vi "GetProcessInstanceRef.vi"(8 "error in (no error)":errorcluster, 10 "Process Name":string, 11 "JKI SMO in":refnum<class "JKI SMO.lvclass">) -> (0 "error out":errorcluster, 2 "Process VI Refnum":refnum<vi>, 3 "JKI SMO out":refnum<class "JKI SMO.lvclass">)   [LabVIEW 2013, in "JKI SMO.lvclass"]
doc: "This method will lookup (and return) the instance reference of <b>Process Name</b>.\n\n---------------------------------------------------------------\nJKI State Machine Objects™\nhttp://jki.net/state-machine-objects/\nCopyright (C) 2005-2015, JKI <info@jki.net>\nALL RIGHTS RESERVED"
uses:
  JKI SMO.lvclass
  JKI SMO.lvclass/JKI SMO.ctl
panel:
  # "For instructions on how to use the JKI State Machine Objects, examples and video tutorials, visit:\nhttp://jki.net/state-machine-objects/\n\nJKI State Machine Objects™\nhttp://jki.net/state-machine-objects/\nCopyright (C) 2005-2015, JKI <info@jki.net>\nALL RIGHTS RESERVED"
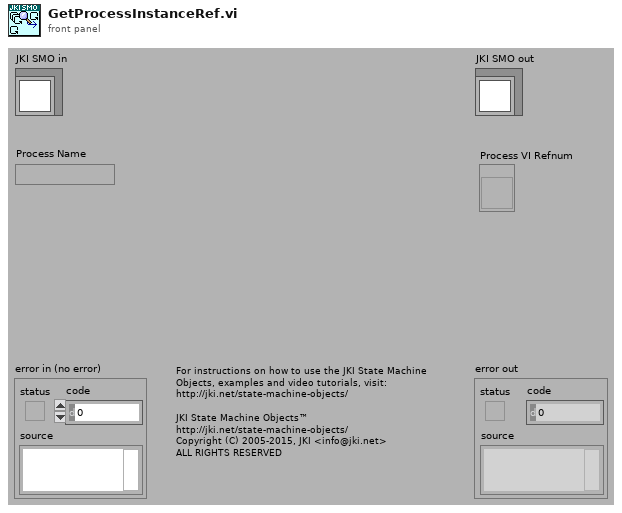
[diagram p1: front panel]
types:
  T1 = typedef "JKI SMO.lvclass/PrivateData--Cluster.ctl" = cluster{"Processes Clone VI Ref [ ]":refnum<vi>[], "Processes Clone Name [ ]":string[], "Process Sync RendezVous":T2, "Protected Events":T3, "Registered Process [ ]":T4[]}
  T2 = typedef "Rendezvous RefNum" = refnum<k1>
  T3 = typedef "JKI SMO.lvclass/ProtectedEvents--Cluster.ctl" = cluster{"StopProcesses":refnum<user-event>, "AbortProcesses":refnum<user-event>}
  T4 = typedef "JKI SMO.lvclass/RegisteredProcessData--Cluster.ctl" = cluster{"Name":string, "Static VI Ref":refnum<vi>}
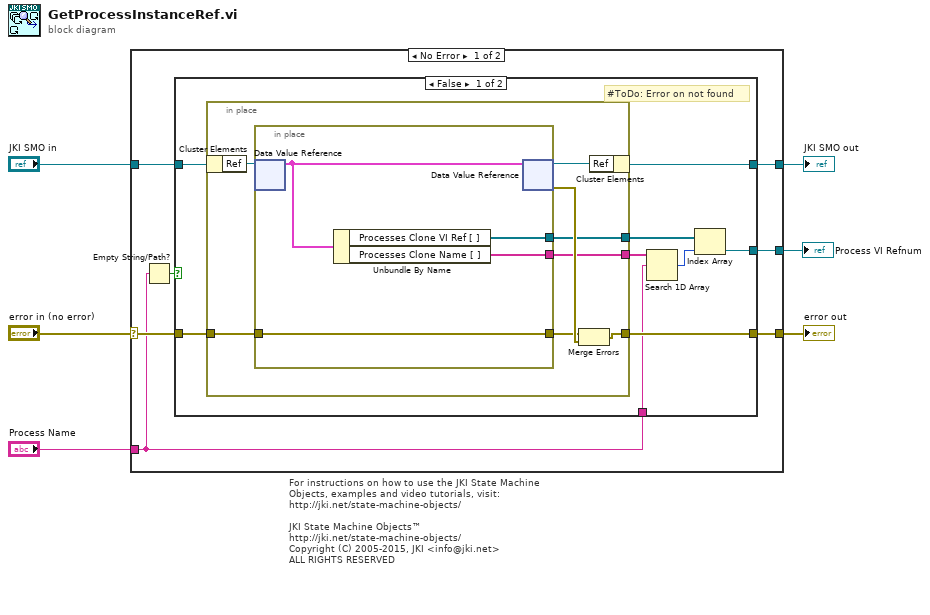
[diagram p0: block diagram]
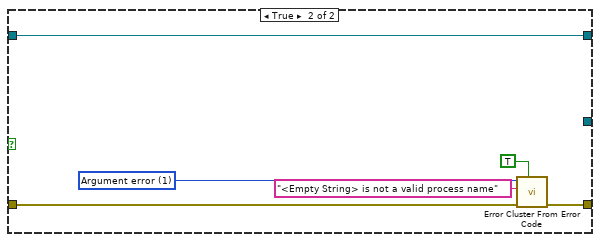
[diagram p2: hidden frame]
diagram:
  # "For instructions on how to use the JKI State Machine Objects, examples and video tutorials, visit:\nhttp://jki.net/state-machine-objects/\n\nJKI State Machine Objects™\nhttp://jki.net/state-machine-objects/\nCopyright (C) 2005-2015, JKI <info@jki.net>\nALL RIGHTS RESERVED"
  n1 = case shown="No Error" "error in (no error)" {
    selector: "error in (no error)" -> [w12 w42]
    tunnel: [w11 w42] -> w5
    tunnel: [w10 w41] -> w3
    tunnel: "JKI SMO in" -> [w13 w41]
    tunnel: [w9 _] -> w2
    tunnel: "Process Name" -> [w7 _]
    frame No Error {
      n2 = Empty String/Path?(string/path=w7) -> (empty?=w8:bool)
      n3 = case shown="False" w8 {
        tunnel: w13 -> [w22 w40]
        tunnel: w12 -> [w21 w38]
        tunnel: [w20 w37] -> w11
        tunnel: [w19 w40] -> w10
        tunnel: [w14 _] -> w9
        tunnel: w7 -> [w17 _]
        frame False {
          # "#ToDo: Error on not found"
          n4 = in-place {
            in-place-border: w21 -> [w29]
            in-place-border: [w26] -> w20
            in-place-border: [w24] -> w15
            in-place-border: [w23] -> w18
            n5 = in-place-cluster #1(w22) -> ("Ref"=w30:refnum<data-value>)
            n6 = in-place {
              in-place-border: w29 -> [w33]
              in-place-border: [w33] -> w27
              in-place-border: [w32] -> w24
              in-place-border: [w31] -> w23
              n7 = in-place-dvr #2(w30) -> (w34:T1)  [unwired: 1 out]
              n8 = Unbundle By Name(w34) -> ("Processes Clone VI Ref [ ]"=w32:refnum<vi>[], "Processes Clone Name [ ]"=w31:string[])
              n9 = in-place-dvr #2(w34) -> (w25:refnum<data-value>, w28:errorcluster)
            }
            n10 = Merge Errors(w27, w28) -> (w26:errorcluster)
            n11 = in-place-cluster #1("Ref"=w25) -> (w19:refnum<class "JKI SMO.lvclass">)
          }
          n12 = Search 1D Array(1D array=w18, element=w17) -> (index of element=w16:i32)  [unwired: 1 in]
          n13 = Index Array(array=w15, index=w16) -> (element=w14:refnum<vi>)
        }
        frame True {
          w39 = 1 items=["No error", "Argument error", "Memory is full", "Out of zone", "End of file", "File already open", "Generic file I/O error", "File not found", "File permission error", "Disk is full", "Duplicate path", "Too many files open", "System feature not enabled", "Resource file not found", "Cannot add resource", "Resource not found", "Image not found", "Image memory error", "Pen does not exist", "Config type invalid", "Config token not found", "Config parse error", "Config memory error", "Bad external code format", "Bad external code offset", "External code not present", "Null window", "Destroy window error", "Null menu", "Print aborted", "Bad print record", "Print driver error", "Windows error during printing", "Memory error during printing", "Print dialog error", "Generic print error", "Invalid device refnum", "Device not found", "Device parameter error", "Device unit error", "Cannot open device", "Device call aborted", "Generic error", "Cancelled by user", "Object ID too low", "Object ID too high", "Object not in heap", "Unknown heap", "Unknown object (invalid DefProc)", "Unknown object (DefProc not in table)", "Message out of range", "Invalid (null) method", "Unknown message", "Manager call not supported", "Bad address", "Network operation in progress", "Network operation timed out", "Connection is busy", "Network attribute not supported", "Network error", "Address in use", "System out of memory", "Connection aborted", "Connection refused", "Not connected", "Already connected", "Connection closed", "Initialization error (interapplication manager)", "Bad occurrence", "Wait on unbound occurrence handler", "Occurrence queue overflow", "Datalog type conflict", "Unused", "Unrecognized type (interapplication manager)", "Memory corrupt", "Failed to make temporary DLL", "Old CIN version", "Drag socket not found", "Failed to load drop-object", "Failed to register OLE object", "Failed to release OLE object", "Format specifier type mismatch", "Unknown format specifier", "Too few format specifiers", "Too many format specifiers", "Scan failed", "Newer CIN version", "Error converting to variant", "Runtime menu error", "Password tampered", "Variant attribute not found", "Incompatible variant data type", "Event data is not available", "Event Store is not present", "Occurrence is not found", "Event Queue is not created", "Event info is not available", "Refnum passed is NULL", "Error retrieving Class GUID", "Error retrieving CoClass GUID", "Error retrieving TypeLib GUID.", "Bad built application magic bytes.", "Specific driver is different from the specific driver associated with the Logical Name.", "There is no session opened to the class driver.", "Max Error", "MAX - Error with config objects", "MAX - Error loading configuration", "MAX - Group not supported"]
          n14 = call <vilib>:"Error Cluster From Error Code.vi"("show call chain? (False)"=TRUE, "error in (no error)"=w38, "error message (\"\")"="<Empty String> is not a valid process name" ("error message (\"\")"), "error code (0)"=w39) -> ("error out"=w37:errorcluster)  [unwired: 5 in]
        }
      }
    }
    frame Error {
    }
  }
  "error out" <- w5
  "JKI SMO out" <- w3
  "Process VI Refnum" <- w2
